vi "FTW-Actor-LocalMessage-Worker.vi"(0 "FTW-ActorInstance In":refnum<class "FTW-ActorInstance.lvclass">, 5 "Message Header":string, 7 "Message Body":string, 9 "Send Rate":dbl, 11 "error in":errorcluster, 12 "Lossless (F)":bool, 13 "Refresh Rate":u32=10 caption="Refresh Rate (10 ms)" format="%d ms") -> (15 "error out":errorcluster)   [LabVIEW 2013, in "FTW-ActorInstance.lvclass"]
uses:
  FTW-ActorInstance.lvclass
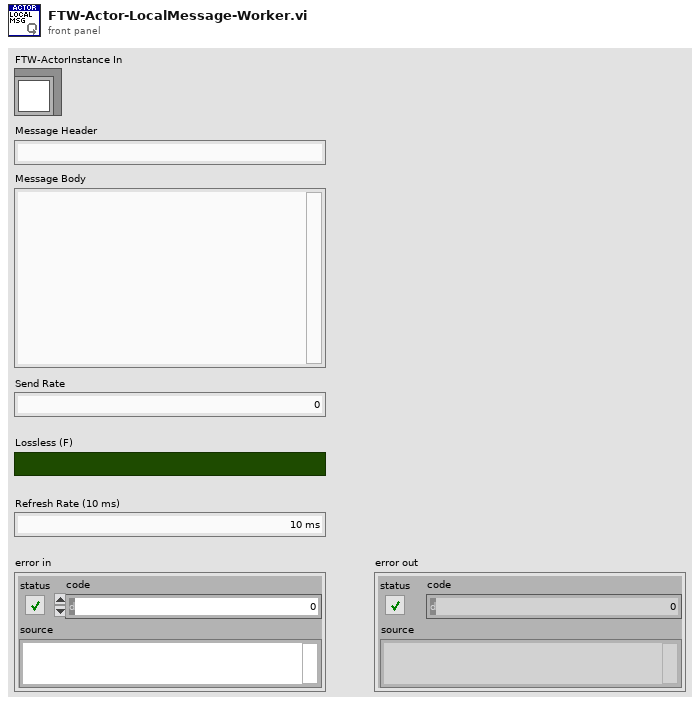
[diagram p1: front panel]
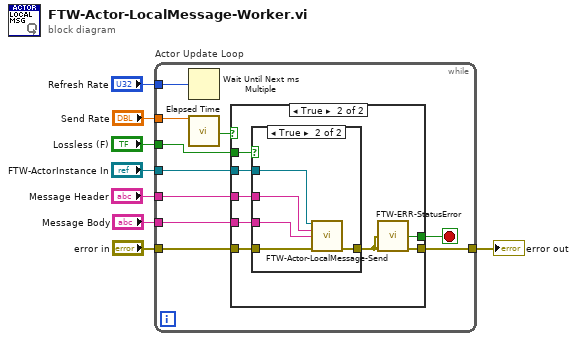
[diagram p0: block diagram]
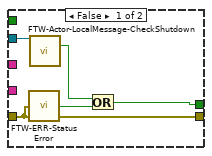
[diagram p2: hidden frame]
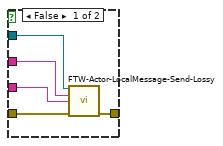
[diagram p3: hidden frame]
diagram:
  n1 = while "Actor Update Loop" {
    tunnel: "FTW-ActorInstance In" -> [w18]
    tunnel: "Message Header" -> [w15]
    tunnel: "Message Body" -> [w14]
    tunnel: "Send Rate" -> [w13]
    tunnel: "Refresh Rate" -> [w12]
    tunnel: "error in" -> [w11]
    tunnel: "Lossless (F)" -> [w9]
    tunnel: [w10] -> w1
    stop <- w17 stop-if-true
    n2 = Wait Until Next ms Multiple(millisecond multiple=w12) -> ()  [unwired: 1 out]
    n3 = call "Elapsed Time"("Time Target (s)"=w13) -> ("Time has Elapsed"=w16:bool)  [unwired: 11 in, 7 out]
    n4 = case shown="True" w16 {
      tunnel: w18 -> [w23 w30]
      tunnel: [w21 w29] -> w17
      tunnel: w15 -> [_ w28]
      tunnel: w14 -> [_ w27]
      tunnel: w11 -> [w19 w26]
      tunnel: [w19 w25] -> w10
      tunnel: w9 -> [_ w24]
      frame False {
        n5 = call "FTW-ERR-StatusError.vi"("error to check"=w19) -> ("Error?"=w20:bool)
        n6 = call "FTW-Actor-LocalMessage-CheckShutdown.vi"("FTW-ActorInstance In"=w23) -> ("Shutdown"=w22:bool)  [unwired: 14 in]
        n7 = Or(x=w22, y=w20) -> (x .or. y?=w21:bool)
      }
      frame True {
        n8 = case shown="True" w24 {
          tunnel: w30 -> [w35 w38]
          tunnel: [w34 w39] -> w25
          tunnel: w28 -> [w33 w37]
          tunnel: w27 -> [w32 w36]
          tunnel: w26 -> [w31 w40]
          frame False {
            n9 = call "FTW-Actor-LocalMessage-Send-Lossy.vi"("FTW-ActorInstance In"=w35, "Message Header"=w33, "Message Body"=w32, "error in"=w31) -> ("error out"=w34:errorcluster)  [unwired: 11 in]
          }
          frame True {
            n10 = call "FTW-Actor-LocalMessage-Send.vi"("FTW-ActorInstance In"=w38, "Message Header"=w37, "Message Body"=w36, "error in"=w40) -> ("error out"=w39:errorcluster)  [unwired: 11 in]
          }
        }
        n11 = call "FTW-ERR-StatusError.vi"("error to check"=w25) -> ("Error?"=w29:bool)
      }
    }
  }
  "error out" <- w1
